vi "inital_VI.vi"() -> ()   [LabVIEW 2024]
uses:
  <vilib>/Analysis/NI_AALPro.lvlib
  <vilib>/Analysis/5stat.llb/RMS (DBL).vi
panel:
  in  "?":enum32{"CONTROLS"}(tab)
  in  "?":bool
  out "SPEED IN RMS":dbl
  out "Phase R":dbl format="%0.2f"
  out "Phase Y":dbl format="%0.2f"
  out "Phase B":dbl format="%0.2f"
  out "Phase R":dbl format="%0.2f"
  out "Phase Y":dbl format="%0.2f"
  out "Phase B":dbl format="%0.2f"
  # "RMS VALUES"
  # "VOLTAGE"
  # "CURRENT"
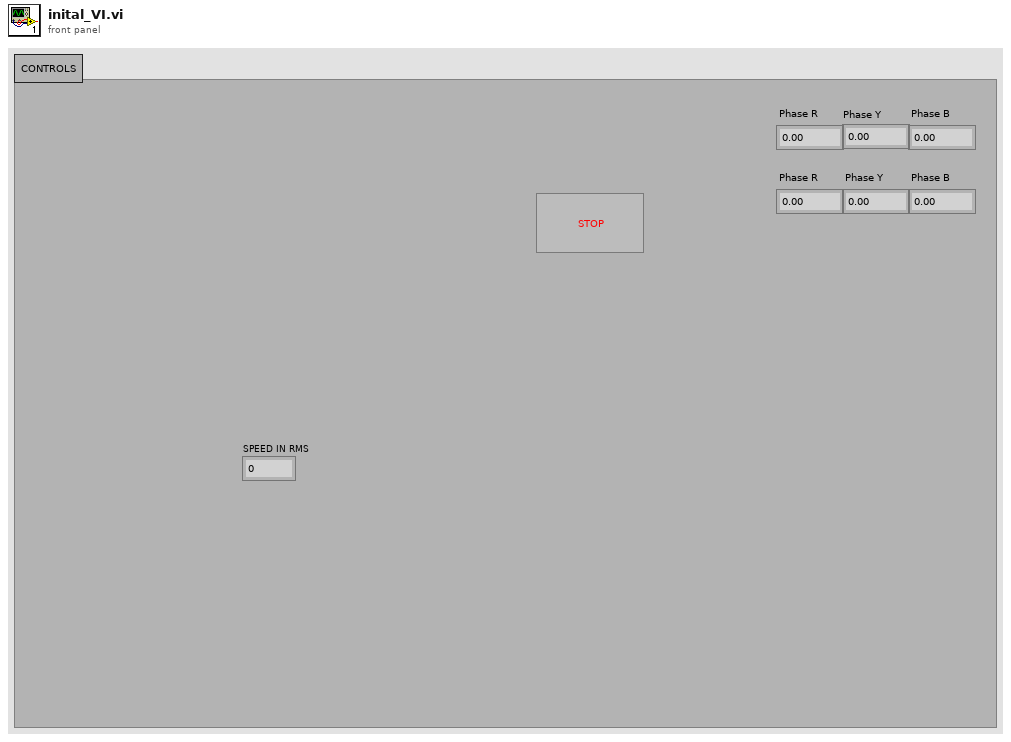
[diagram p1: front panel]
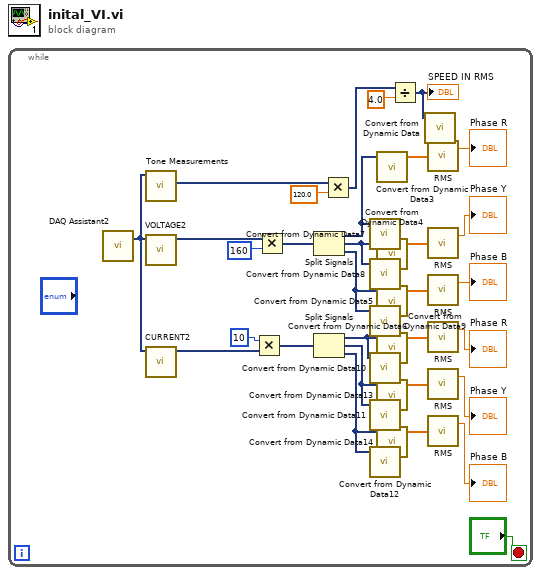
[diagram p0: block diagram]
diagram:
  n1 = while {
    stop <- "?" stop-if-true
    n2 = call "DAQ Assistant2"() -> ("data"=w25:dynamicdata)  [unwired: 16 in, 3 out]
    n3 = call "Tone Measurements"("Signals"=w25) -> ("Frequency"=w23:dynamicdata)  [unwired: 9 in, 1 out]
    n4 = call "VOLTAGE2"("Signals"=w25) -> ("Signal Out"=w29:dynamicdata)  [unwired: 9 in, 1 out]
    n5 = call "CURRENT2"("Signals"=w25) -> ("Signal Out"=w27:dynamicdata)  [unwired: 9 in, 1 out]
    n6 = Multiply(x=10, y=w27) -> (x*y=w20:dynamicdata)
    n7 = Multiply(x=w29, y=160) -> (x*y=w26:dynamicdata)
    n8 = Split Signals(w26) -> (w19:dynamicdata, w16:dynamicdata, w13:dynamicdata)  [unwired: 3 in]
    n9 = Split Signals(w20) -> (w4:dynamicdata, w3:dynamicdata, w2:dynamicdata)  [unwired: 3 in]
    n10 = Multiply(x=w23, y=120.0) -> (x*y=w22:dynamicdata)
    n11 = call "Convert from Dynamic Data7"("Dynamic Data Type"=w19) -> ()  [unwired: 3 in, 1 out]
    n12 = call "Convert from Dynamic Data8"("Dynamic Data Type"=w16) -> ()  [unwired: 3 in, 1 out]
    n13 = call "Convert from Dynamic Data9"("Dynamic Data Type"=w13) -> ()  [unwired: 3 in, 1 out]
    n14 = call "Convert from Dynamic Data10"("Dynamic Data Type"=w4) -> ()  [unwired: 3 in, 1 out]
    n15 = call "Convert from Dynamic Data11"("Dynamic Data Type"=w3) -> ()  [unwired: 3 in, 1 out]
    n16 = call "Convert from Dynamic Data12"("Dynamic Data Type"=w2) -> ()  [unwired: 3 in, 1 out]
    n17 = call "Convert from Dynamic Data3"("Dynamic Data Type"=w19) -> ("Array"=w18:dbl[])  [unwired: 3 in]
    n18 = call "Convert from Dynamic Data4"("Dynamic Data Type"=w16) -> ("Array"=w15:dbl[])  [unwired: 3 in]
    n19 = call "Convert from Dynamic Data5"("Dynamic Data Type"=w13) -> ("Array"=w12:dbl[])  [unwired: 3 in]
    n20 = call "Convert from Dynamic Data6"("Dynamic Data Type"=w4) -> ("Array"=w10:dbl[])  [unwired: 3 in]
    n21 = call "Convert from Dynamic Data13"("Dynamic Data Type"=w3) -> ("Array"=w8:dbl[])  [unwired: 3 in]
    n22 = call "Convert from Dynamic Data14"("Dynamic Data Type"=w2) -> ("Array"=w6:dbl[])  [unwired: 3 in]
    n23 = Divide(x=w22, y=4.0) -> (x/y=w21:dynamicdata)
    "SPEED IN RMS" <- w21
    n24 = call "Convert from Dynamic Data"("Dynamic Data Type"=w21) -> ()  [unwired: 3 in, 1 out]
    n25 = call-poly <vilib>:"RMS.vi"("X"=w18) -> ("rms value"=→"Phase R":dbl)  [unwired: 1 out]
    n26 = call-poly <vilib>:"RMS.vi"("X"=w15) -> ("rms value"=→"Phase Y":dbl)  [unwired: 1 out]
    n27 = call-poly <vilib>:"RMS.vi"("X"=w12) -> ("rms value"=→"Phase B":dbl)  [unwired: 1 out]
    n28 = call-poly <vilib>:"RMS.vi"("X"=w10) -> ("rms value"=→"Phase R":dbl)  [unwired: 1 out]
    n29 = call-poly <vilib>:"RMS.vi"("X"=w8) -> ("rms value"=→"Phase Y":dbl)  [unwired: 1 out]
    n30 = call-poly <vilib>:"RMS.vi"("X"=w6) -> ("rms value"=→"Phase B":dbl)  [unwired: 1 out]
  }
